vi "Launcher.vi"() -> ()   [LabVIEW 2019]
uses:
  Main GUI/Main GUI/Main GUI.lvclass
  C:/Program Files (x86)/National Instruments/LabVIEW 2019/vi.lib/ActorFramework/Actor/Actor.lvclass
  <vilib>/ActorFramework/Actor/Actor.lvclass
panel:
  out "error out":errorcluster
  in  "error in (no error)":errorcluster
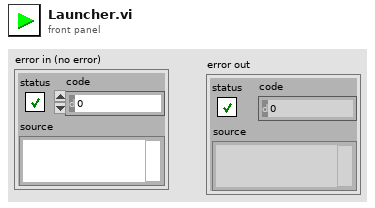
[diagram p1: front panel]
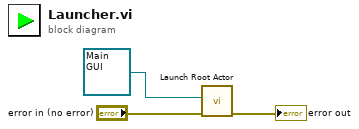
[diagram p0: block diagram]
diagram:
  n1 = call <vilib>:"Launch Root Actor.vi"("error in (no error)"="error in (no error)", "Actor"=refnum<class "Main GUI.lvclass"> refnum ("Main GUI.lvlib:Main GUI.lvclass")) -> ("error out"=→"error out":errorcluster)  [unwired: 8 in, 1 out]
